vi "save_config_file.vi"(8 "error in (no error)":errorcluster, 9 "config cluster variant":variant, 11 "DAQmxWriteSignals in":refnum<class "SignalWriterDL090202DAQmx.lvclass">) -> (0 "error out":errorcluster, 3 "DAQmxWriteSignals out":refnum<class "SignalWriterDL090202DAQmx.lvclass">)   [LabVIEW 2010]
uses:
  SignalWriterDL090202DAQmx.lvclass
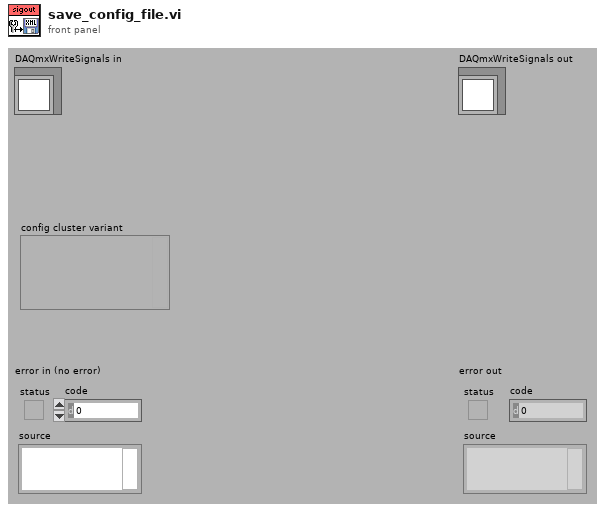
[diagram p1: front panel]
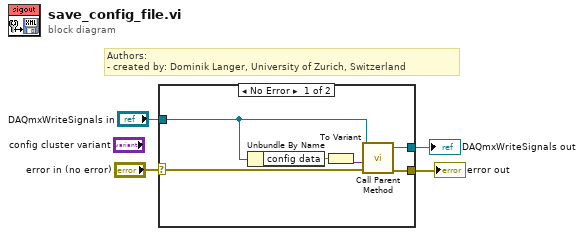
[diagram p0: block diagram]
diagram:
  # "Authors: \n- created by: Dominik Langer, University of Zurich, Switzerland"
  n1 = case shown="No Error" "error in (no error)" {
    selector: "error in (no error)" -> [w6 w12]
    tunnel: "DAQmxWriteSignals in" -> [w5 w11]
    tunnel: [w7 w11] -> w3
    tunnel: [w8 w12] -> w2
    frame No Error {
      n2 = Unbundle By Name(w5) -> ("config data"=w10)
      n3 = To Variant(anything=w10) -> (Variant=w9:variant)
      n4 = call-parent "Call Parent Method"("error in (no error)"=w6, "config cluster variant"=w9, "GenericPlugin in"=w5) -> ("error out"=w8:errorcluster, "GenericPlugin out"=w7:refnum<class "SignalWriterDL090202DAQmx.lvclass">)  [unwired: 1 in, 6 out]
    }
    frame Error {
    }
  }
  "error out" <- w2
  "DAQmxWriteSignals out" <- w3
